vi "Enqueue Data To Nodes.vi"(8 "error in":errorcluster, 9 "Input Valid":bool, 10 "Input Data":T1, 11 "Communication FIFOs":T2) -> (0 "error out":errorcluster, 1 "Send Success?":bool, 4 "Ready for Input":bool)   [LabVIEW 2014, in "IO Node Logic Template.lvlib"]
uses:
  IO Node Logic Template.lvlib
  Controls/All Nodes Resources.ctl
  Node/Controls/NodeResources FIFOs.ctl
  <vilib>/SPI API/SPIAPI/Controls/SPI Response Information.ctl
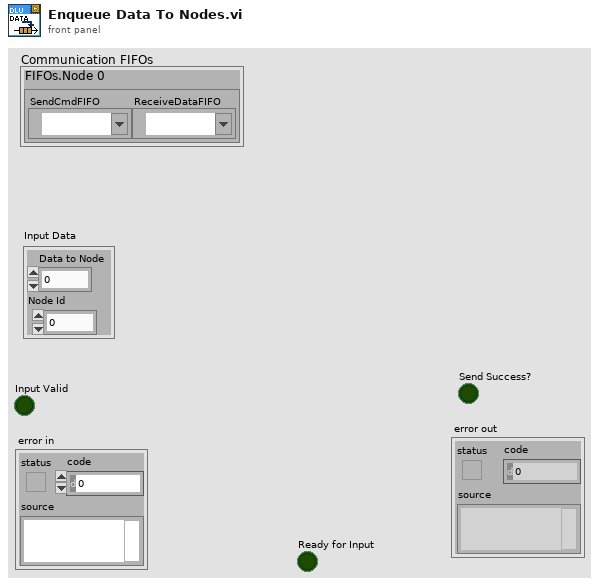
[diagram p1: front panel]
types:
  T1 = typedef "SPI Response Information.ctl" = cluster{"Data to Node":u64, "Node Id":u16}
  T2 = typedef "IO Node Logic Template.lvlib/All Nodes Resources.ctl" = cluster{"FIFOs.Node 0":T3}
  T3 = typedef "IO Node Logic Template.lvlib/NodeResources FIFOs.ctl" = cluster{"SendCmdFIFO":refnum<k21>, "ReceiveDataFIFO":refnum<k21>}
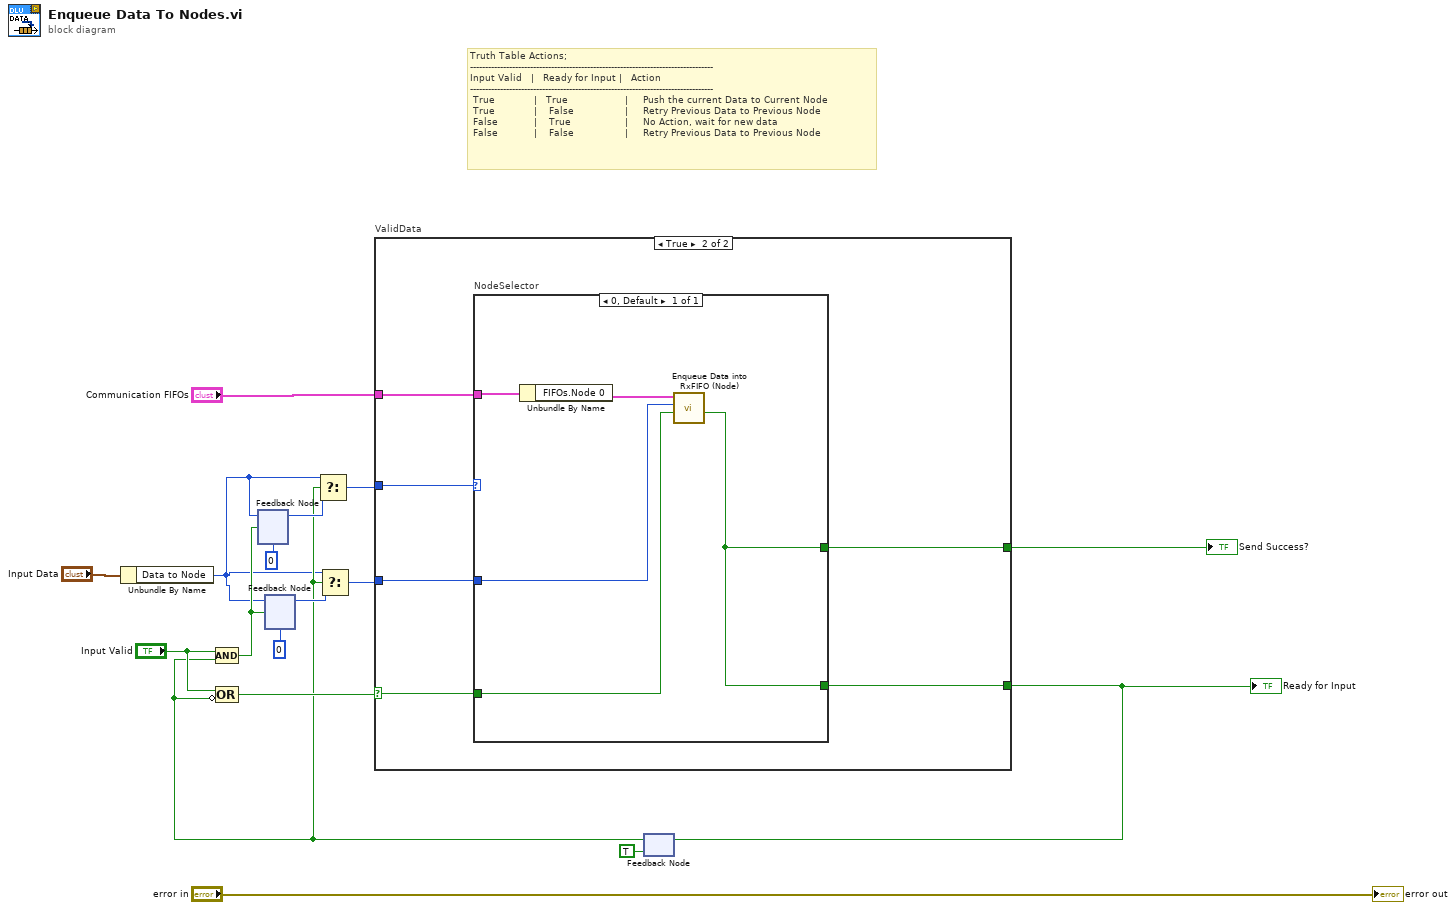
[diagram p0: block diagram]
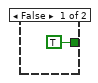
[diagram p2: hidden frame]
diagram:
  # "Truth Table Actions;\n---------------------------------------------------------------------------------\nInput Valid   |   Ready for Input |   Action\n---------------------------------------------------------------------------------\n True             |   True                   |     Push the current Data to Current Node\n True             |    False                 |     Retry Previous Data to Previous Node\n False            |    True                  |     No Action, wait for new data\n False            |    False                 |     Retry Previous Data to Previous Node"
  n1 = Unbundle By Name("Input Data") -> ("Data to Node"=w1:u64)
  n2 = feedback #1(u8 0 ("Current Node")) -> (w10:u64)
  n3 = feedback #2(u64 0 ("Input Data")) -> (w8:u64)
  n4 = feedback #3(TRUE ("Send Success?")) -> (w6:bool)
  n5 = Compound Arithmetic op=AND("Input Valid", w6) -> (w14:bool)
  n6 = Compound Arithmetic op=OR("Input Valid", invert w6) -> (w12:bool)
  n7 = feedback-in #1(w1, w14) -> ()
  n8 = feedback-in #2(w1, w14) -> ()
  n9 = Select(t=w1, s=w6, f=w10) -> (s? t:f=w11:u64)
  n10 = Select(t=w1, s=w6, f=w8) -> (s? t:f=w9:u64)
  n11 = case "ValidData" shown="True" w12 {
    selector: w12 -> [_ w21]
    tunnel: "Communication FIFOs" -> [_ w24]
    tunnel: w11 -> [_ w23]
    tunnel: w9 -> [_ w22]
    tunnel: [TRUE ("Send Success?") w20] -> w15
    tunnel: [_ w19] -> w2
    frame False {
    }
    frame True {
      n12 = case "NodeSelector" shown="0, Default" w23 {
        tunnel: w24 -> [w29]
        tunnel: w22 -> [w27]
        tunnel: w21 -> [w26]
        tunnel: [w25] -> w20
        tunnel: [w25] -> w19
        frame 0, Default {
          n13 = Unbundle By Name(w29) -> ("FIFOs.Node 0"=w28:T3)
          n14 = call "Enqueue Data into RxFIFO (Node).vi"("Input Valid"=w26, "Input Data"=w27, "FIFOs: I/O Node"=w28) -> ("Send Success?"=w25:bool)  [unwired: 6 in, 2 out]
        }
      }
    }
  }
  "Ready for Input" <- w15
  "Send Success?" <- w2
  n15 = feedback-in #3(w15) -> ()
  "error out" <- "error in"
